vi "Launcher.vi"() -> ()   [LabVIEW 2014]
uses:
  Target/Target/Target.lvclass
  Proxy/Proxy/Proxy.lvclass
  Proxy/Proxy/Proxy.lvclass/Proxy.ctl
  <vilib>/ActorFramework/Stop Msg/Stop Msg.lvclass/Stop Msg.ctl
  <vilib>/ActorFramework/Message Enqueuer/Message Enqueuer.lvclass/Message Enqueuer.ctl
  Proxy/Proxy/Write Target Enq.vi
  <vilib>/ActorFramework/Stop Msg/Send Emergency Stop.vi
  <vilib>/ActorFramework/Stop Msg/Send Normal Stop.vi
  <vilib>/ActorFramework/Message Enqueuer/Enqueue.vi
  <vilib>/ActorFramework/Message Enqueuer/Enqueue Critical.vi
  <vilib>/ActorFramework/Message Priority Queue/Priority Enqueue.vi
  <vilib>/ActorFramework/Stop Msg/Stop Msg.lvclass
  Target/Target Messages/Action Msg/Action Msg.lvclass
  Source Actor/Source Actor Messages/Source Action Msg/Source Action Msg.lvclass
  Proxy/Proxy Messages/Proxy Action Msg/Proxy Action Msg.lvclass
  <vilib>/ActorFramework/Actor/Actor.lvclass
  <vilib>/ActorFramework/Reply Msg/Reply Msg.lvclass
  Target/Get Proxy Enq Msg.lvclass
  <vilib>/ActorFramework/Message Enqueuer/Message Enqueuer.lvclass
panel:
  out "error out":errorcluster
  in  "unsupported MSG":bool
  in  "Send target msg via proxy":bool
  in  "final error code":i32
  in  "Send proxy msg":bool
  in  "Send target msg direct":bool
  in  "Stop":bool
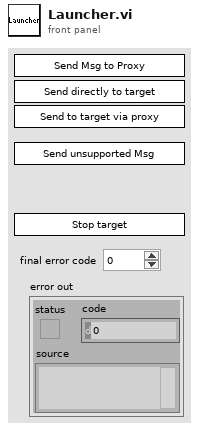
[diagram p1: front panel]
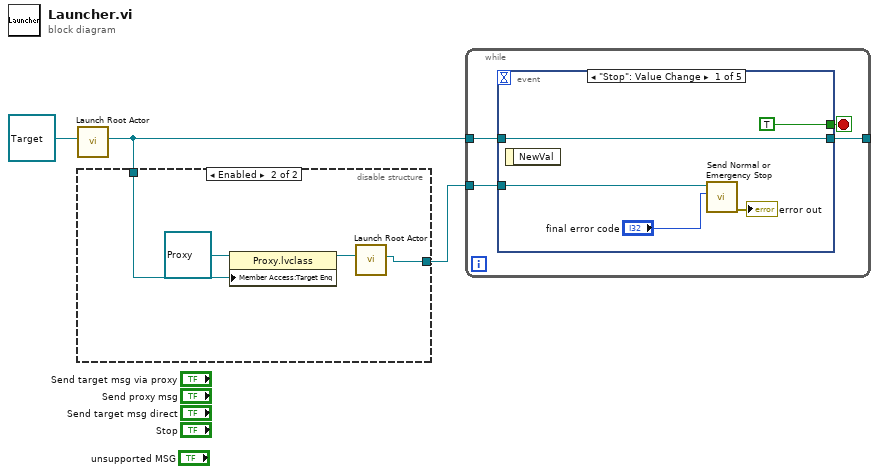
[diagram p0: block diagram]
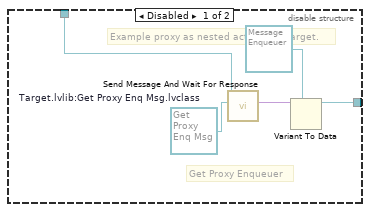
[diagram p2: hidden frame]
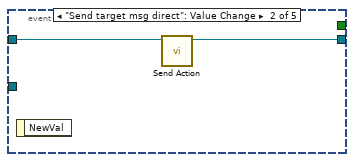
[diagram p3: hidden frame]
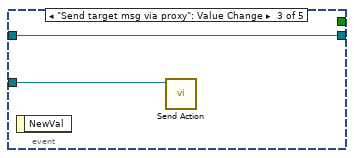
[diagram p4: hidden frame]
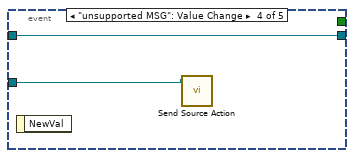
[diagram p5: hidden frame]
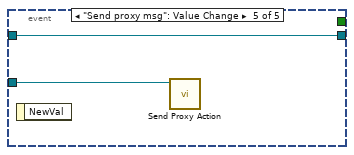
[diagram p6: hidden frame]
diagram:
  n1 = call <vilib>:"Launch Root Actor.vi"("Actor"=refnum<class "Target.lvclass"> refnum ("Target.lvlib:Target.lvclass")) -> ("Actor's Enqueuer"=w2:refnum<class "Message Enqueuer.lvclass">)  [unwired: 9 in, 1 out]
  n2 = disable-structure shown="Enabled" {
    disable-tunnel: w2 -> [w8 w10]
    disable-tunnel: [w5 w9] -> w1
    frame Disabled {
      w7 = refnum<class "Get Proxy Enq Msg.lvclass"> refnum  # Target.lvlib:Get Proxy Enq Msg.lvclass
      # "Example proxy as nested actor from target."
      # "Get Proxy Enqueuer"
      n3 = call <vilib>:"Send Message And Wait For Response.vi"("Original Message"=w7, "Message Enqueuer in"=w8) -> ("Reply"=w6:variant)  [unwired: 6 in, 3 out]
      n4 = Variant To Data(type=refnum<class "Message Enqueuer.lvclass"> refnum ("Target Enq"), Variant=w6) -> (data=w5:refnum<class "Message Enqueuer.lvclass">)  [unwired: 1 in, 1 out]
    }
    frame Enabled {
      n5 = property class="Proxy.lvclass"(reference=refnum<class "Proxy.lvclass"> refnum ("Proxy.lvlib:Proxy.lvclass"), "Member Access:Target Enq"=w10) -> (reference out=w11:refnum<class "Proxy.lvclass">)  [unwired: 1 in, 1 out]
      n6 = call <vilib>:"Launch Root Actor.vi"("Actor"=w11) -> ("Actor's Enqueuer"=w9:refnum<class "Message Enqueuer.lvclass">)  [unwired: 9 in, 1 out]
    }
  }
  n7 = while {
    tunnel: w2 -> [w15]
    tunnel: [w14] -> _
    tunnel: w1 -> [w13]
    stop <- w16 stop-if-true
    n8 = event shown="[0] \"Stop\": Value Change" {
      selector: _ -> [_ _ _ _ _]
      dyn-events: _ -> [_ _ _ _ _]
      timeout: _ -> [_ _ _ _ _]
      tunnel: [TRUE _ _ _ _] -> w16
      tunnel: w15 -> [w20 w23 w24 w27 w28]
      tunnel: [w20 w22 w24 w27 w28] -> w14
      tunnel: w13 -> [w19 _ w25 w26 w29]
      event "Stop": Value Change {
        n9 = event-data() -> ()  [unwired: 1 in, 1 out]
        n10 = call <vilib>:"Send Normal or Emergency Stop.vi"("final error code"="final error code", "Message Enqueuer"=w19) -> ("error out"=→"error out":errorcluster)  [unwired: 9 in]
      }
      event "Send target msg direct": Value Change {
        n11 = event-data() -> ()  [unwired: 1 in, 1 out]
        n12 = call "Send Action.vi"("Message Enqueuer"=w23) -> ("Message Enqueuer out"=w22:refnum<class "Message Enqueuer.lvclass">)  [unwired: 9 in, 1 out]
      }
      event "Send target msg via proxy": Value Change {
        n13 = event-data() -> ()  [unwired: 1 in, 1 out]
        n14 = call "Send Action.vi"("Message Enqueuer"=w25) -> ()  [unwired: 9 in, 2 out]
      }
      event "unsupported MSG": Value Change {
        n15 = event-data() -> ()  [unwired: 1 in, 1 out]
        n16 = call "Send Source Action.vi"("Message Enqueuer"=w26) -> ()  [unwired: 9 in, 2 out]
      }
      event "Send proxy msg": Value Change {
        n17 = event-data() -> ()  [unwired: 1 in, 1 out]
        n18 = call "Send Proxy Action.vi"("Message Enqueuer"=w29) -> ()  [unwired: 9 in, 2 out]
      }
    }
  }
